vi "FirstNumber.vi"(0 "Input String":string="OptCernox1010X4981.cal2") -> (1 "Number Stings":string[](array[string])=["1010", "4981", "2"], 2 "Numbers":ext[](array[numeric])=[1010.0, 4981.0, 2.0] format="%.2f", 3 "FirstNumber":string="1010", 4 "LastNumber":string="2", 5 "FirstNumber":ext=1010.0 format="%.2f", 6 "LastNumber":ext=2.0 format="%.2f")   [LabVIEW 2025]
doc: "Author: Scott Hannahs <sth@magnet.fsu.edu>\n\nThis software is licensed for use under the “MIT License\"\nCopyright (c) 2025 Scott Hannahs, sth@sth@magnet.sthnet.net\n\nPermission is hereby granted, free of charge, to any person obtaining a copy of this software and associated documentation files (the \"Software\"), to deal in the Software without restriction, including without limitation the rights to use, copy, modify, merge, publish, distribute, sublicense, and/or sell copies of the Software, and to permit persons to whom the Software is furnished to do so, subject to the following conditions: The above copyright notice and this permission notice shall be included in all copies or substantial portions of the Software.\n\nTHE SOFTWARE IS PROVIDED \"AS IS\", WITHOUT WARRANTY OF ANY KIND, EXPRESS OR IMPLIED, INCLUDING BUT NOT LIMITED TO THE WARRANTIES OF MERCHANTABILITY, FITNESS FOR A PARTICULAR PURPOSE AND NONINFRINGEMENT. IN NO EVENT SHALL THE AUTHORS OR COPYRIGHT HOLDERS BE LIABLE FOR ANY CLAIM, DAMAGES OR OTHER LIABILITY, WHETHER IN AN ACTION OF CONTRACT, TORT OR OTHERWISE, ARISING FROM, OUT OF OR IN CONNECTION WITH THE SOFTWARE OR THE USE OR OTHER DEALINGS IN THE SOFTWARE."
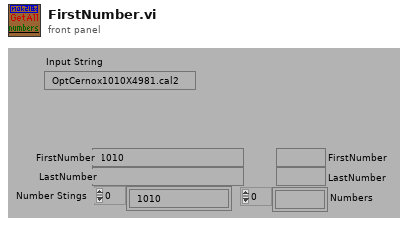
[diagram p1: front panel]
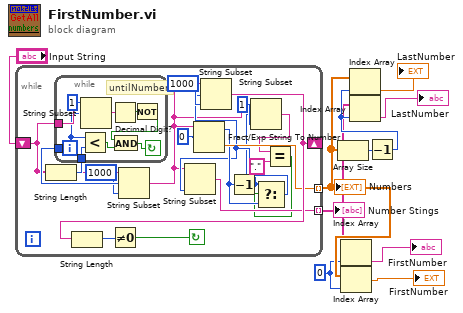
[diagram p0: block diagram]
diagram:
  w5 = 0
  n1 = while {
    tunnel: [w19] -> w7 mode=indexing
    tunnel: [w21] -> w6 mode=indexing
    shift-left: "Input String" -> [w25]
    shift-right: [w24] -> _
    stop <- w22 continue-if-true
    n2 = String Length(string=w25) -> (length=w27:i32)
    n3 = while {
      tunnel: [w30] -> w28
      tunnel: w27 -> [w35]
      tunnel: w25 -> [w37]
      i -> [w30]
      stop <- w32 continue-if-true
      # "untilNumber"
      n4 = Less?(x=w30, y=w35) -> (x < y?=w36:bool)
      n5 = String Subset(string=w37, offset (0)=w30, length (rest)=1) -> (substring=w34:string)
      n6 = Decimal Digit?(1:w34) -> (0:w33:bool)
      n7 = Not(x=w33) -> (.not. x?=w31:bool)
      n8 = And(x=w31, y=w36) -> (x .and. y?=w32:bool)
    }
    n9 = String Subset(string=w25, offset (0)=w28, length (rest)=1000) -> (substring=w12:string)
    n10 = Fract/Exp String To Number(string=w12, offset=0) -> (offset past number=w15:i32, number=w19:dbl)  [unwired: 2 in]
    n11 = Decrement(x=w15) -> (x-1=w11:i32)
    n12 = String Subset(string=w12, offset (0)=w11, length (rest)=1) -> (substring=w16:string)
    n13 = Equal?(x=w16, y=".") -> (x = y?=w14:bool)
    n14 = Select(t=w11, s=w14, f=w15) -> (s? t:f=w13:i32)
    n15 = String Subset(string=w12, length (rest)=w13) -> (substring=w21:string)  [unwired: 1 in]
    n16 = String Subset(string=w12, offset (0)=w13, length (rest)=1000) -> (substring=w24:string)
    n17 = String Length(string=w24) -> (length=w23:i32)
    n18 = Not Equal To 0?(x=w23) -> (x != 0?=w22:bool)
  }
  "Numbers" <- w7
  "Number Stings" <- w6
  n19 = Array Size(array=w7) -> (size(s)=w9:i32)
  n20 = Index Array(array=w6, index=w5) -> (element=→"FirstNumber":string)
  n21 = Index Array(array=w7, index=w5) -> (element=→"FirstNumber":dbl)
  n22 = Decrement(x=w9) -> (x-1=w8:i32)
  n23 = Index Array(array=w7, index=w8) -> (element=→"LastNumber":dbl)
  n24 = Index Array(array=w6, index=w8) -> (element=→"LastNumber":string)
